vi "testFlushTel.vi"(8 "error in (no error)":errorcluster) -> (0 "error out":errorcluster)   [LabVIEW 2018]
doc: "Test the flushTel.vi."
uses:
  src/TcpServer/TcpServer.lvclass
  src/TcpServer/TcpServer.lvclass/TcpServer.ctl
  src/TcpServerTel/TcpServerTel.lvclass/TcpServerTel.ctl
  <vilib>/addons/_JKI Toolkits/Caraya/classes/Assert/Assert Equal Value_Variant.vi
  src/TcpServerTel/TcpServerTel.lvclass
  <vilib>/addons/_JKI Toolkits/Caraya/classes/Test/Test.lvclass
  <vilib>/addons/_JKI Toolkits/Caraya/classes/Assert/Assert.lvclass
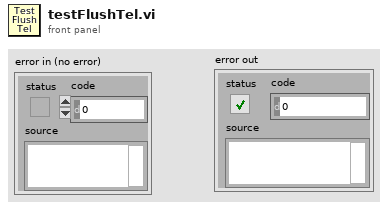
[diagram p1: front panel]
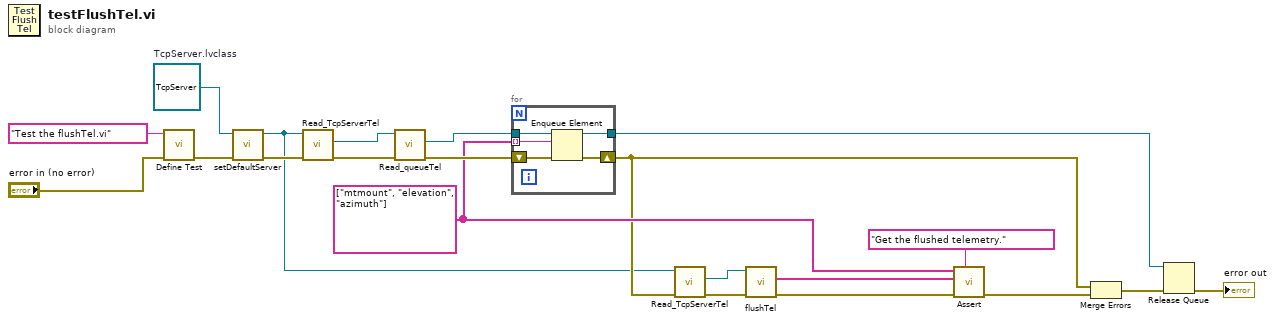
[diagram p0: block diagram]
diagram:
  w6 = string[] ["mtmount", "elevation", "azimuth"]
  w2 = refnum<class "TcpServer.lvclass"> refnum  # TcpServer.lvclass
  n1 = call <vilib>:"Define Test.vi"("error in (no error)"="error in (no error)", "Label (VI Title)"="Test the flushTel.vi") -> ("error out"=w20:errorcluster)  [unwired: 9 in]
  n2 = call "setDefaultServer.vi"("error in (no error)"=w20, "TcpServer.lvclass"=w2) -> ("error out"=w9:errorcluster, "tcpServer out"=w1:refnum<class "TcpServer.lvclass">)  [unwired: 8 in]
  n3 = call "Read_TcpServerTel.vi"("error in (no error)"=w9, "TcpServer in"=w1) -> ("error out"=w15:errorcluster, "TcpServerTel.lvclass"=w16:refnum<class "TcpServerTel.lvclass">)  [unwired: 7 in, 1 out]
  n4 = call "Read_queueTel.vi"("error in (no error)"=w15, "TcpServerTel in"=w16) -> ("error out"=w12:errorcluster, "telQueueServer"=w11:refnum<queue>)  [unwired: 7 in, 1 out]
  n5 = for {
    tunnel: w11 -> [w25]
    tunnel: w6 -> [w24] mode=indexing
    tunnel: [w22] -> w10
    shift-right: [w23] -> w5
    shift-left: w12 -> [w26]
    n6 = Enqueue Element(queue=w25, element=w24, error in (no error)=w26) -> (queue out=w22:refnum<queue>, error out=w23:errorcluster)  [unwired: 1 in, 1 out]
  }
  n7 = call "Read_TcpServerTel.vi"("error in (no error)"=w5, "TcpServer in"=w1) -> ("error out"=w4:errorcluster, "TcpServerTel.lvclass"=w3:refnum<class "TcpServerTel.lvclass">)  [unwired: 7 in, 1 out]
  n8 = call "flushTel.vi"("error in (no error)"=w4, "tcpServerTel in"=w3) -> ("error out"=w8:errorcluster, "telemetry flushed"=w7:string[])  [unwired: 7 in, 1 out]
  n9 = call-poly <vilib>:"Assert.vi"("Label"="Get the flushed telemetry.", "error in (no error)"=w8, "Y"=w7, "X"=w6) -> ("error out"=w17:errorcluster)  [unwired: 7 in]
  n10 = Merge Errors(w5, w17) -> (w13:errorcluster)
  n11 = Release Queue(queue=w10, error in (no error)=w13) -> (error out=→"error out":errorcluster)  [unwired: 1 in, 2 out]
